vi "Calculate rectangle pixels and lines.vi"(8 "No of Z planes":i32=1, 9 "Resolution multiplier":dbl=1.0, 10 "XY Coordinates (zero based)":i32[](array[numeric])) -> (1 "Number of lines (scaled)":dbl, 3 "Pixels in ROI":dbl)   [LabVIEW 2017]
panel:
  # "X start\nY start\nX stop\nY stop"
  # "<--- Automatically switches to output the shortest dimension, assuming that rectangles longer on their Y axis are handled as vertical ROI, meaning that their X dimension becomes the number of lines/miniscans."
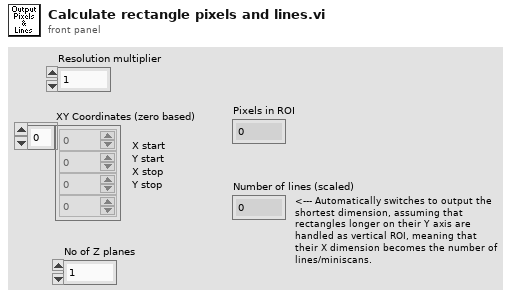
[diagram p1: front panel]
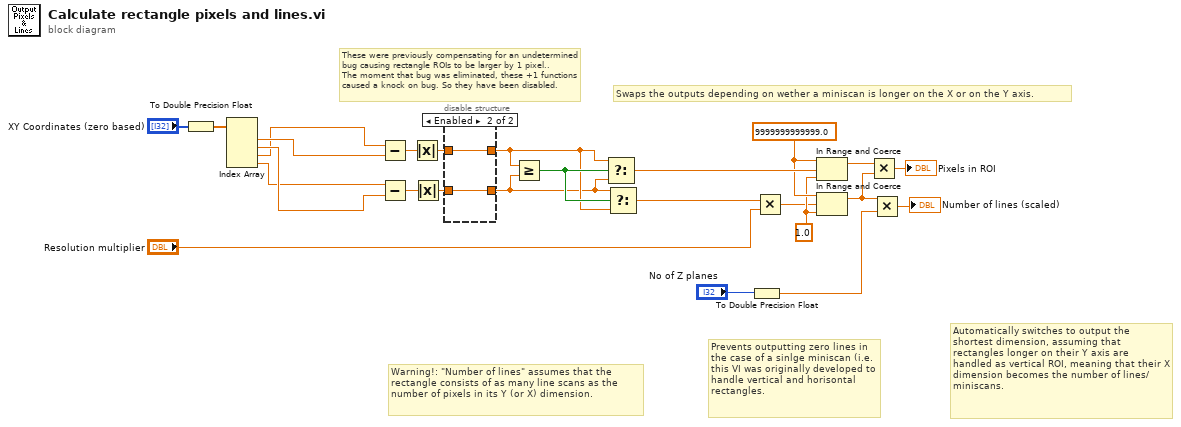
[diagram p0: block diagram]
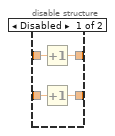
[diagram p2: hidden frame]
diagram:
  w11 = 1.0 ("lower limit")
  w12 = 9999999999999.0 ("upper limit")
  # "These were previously compensating for an undetermined bug causing rectangle ROIs to be larger by 1 pixel..\nThe moment that bug was eliminated, these +1 functions caused a knock on bug. So they have been disabled."
  # "Automatically switches to output the shortest dimension, assuming that rectangles longer on their Y axis are handled as vertical ROI, meaning that their X dimension becomes the number of lines/miniscans."
  # "Prevents outputting zero lines in the case of a sinlge miniscan (i.e. this VI was originally developed to handle vertical and horisontal rectangles."
  # "Warning!: \"Number of lines\" assumes that the rectangle consists of as many line scans as the number of pixels in its Y (or X) dimension."
  # "Swaps the outputs depending on wether a miniscan is longer on the X or on the Y axis."
  n1 = To Double Precision Float(number="XY Coordinates (zero based)") -> (double precision float=w15:dbl[])
  n2 = Index Array(array=w15) -> (element #1=w20:dbl, element #2=w19:dbl, element #3=w18:dbl, element #4=w17:dbl)  [unwired: 4 in]
  n3 = Subtract(x=w18, y=w20) -> (x-y=w24:dbl)
  n4 = Subtract(x=w17, y=w19) -> (x-y=w25:dbl)
  n5 = Absolute Value(x=w24) -> (abs(x)=w23:dbl)
  n6 = Absolute Value(x=w25) -> (abs(x)=w22:dbl)
  n7 = disable-structure shown="Enabled" {
    disable-tunnel: w23 -> [w29 w31]
    disable-tunnel: w22 -> [w28 w30]
    disable-tunnel: [w27 w31] -> w7
    disable-tunnel: [w26 w30] -> w6
    frame Disabled {
      n8 = Increment(x=w29) -> (x+1=w27:dbl)
      n9 = Increment(x=w28) -> (x+1=w26:dbl)
    }
    frame Enabled {
    }
  }
  n10 = Greater Or Equal?(x=w7, y=w6) -> (x >= y?=w21:bool)
  n11 = Select(t=w7, s=w21, f=w6) -> (s? t:f=w14:dbl)
  n12 = Select(t=w6, s=w21, f=w7) -> (s? t:f=w10:dbl)
  n13 = To Double Precision Float(number="No of Z planes") -> (double precision float=w2:dbl)
  n14 = Multiply(x=w10, y="Resolution multiplier") -> (x*y=w9:dbl)
  n15 = In Range and Coerce(upper limit=w12, x=w14, lower limit=w11) -> (coerced(x)=w13:dbl)  [unwired: 1 out]
  n16 = In Range and Coerce(upper limit=w12, x=w9, lower limit=w11) -> (coerced(x)=w3:dbl)  [unwired: 1 out]
  n17 = Multiply(x=w13, y=w3) -> (x*y=→"Pixels in ROI":dbl)
  n18 = Multiply(x=w3, y=w2) -> (x*y=→"Number of lines (scaled)":dbl)
